vi "Sensor.vi"() -> ()   [LabVIEW 2020]
uses:
  Global_Variable/Global.vi
  Global_Variable/excursion.vi
panel:
  in  "Sensor":T1
  # "扭矩偏移"
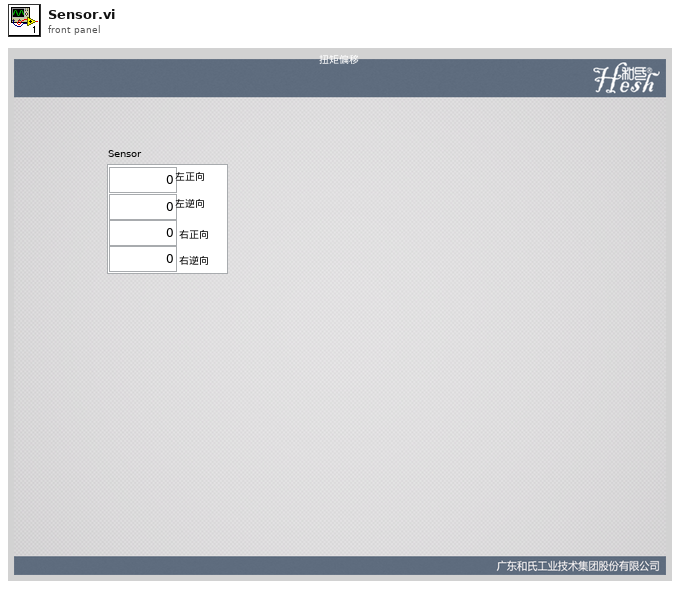
[diagram p1: front panel]
types:
  T1 = cluster{"左正向":dbl, "左逆向":dbl, "右正向":dbl, "右逆向":dbl}
  T2 = typedef "Sensor.ctl" = cluster{"左正向":dbl, "左逆向":dbl, "右正向":dbl, "右逆向":dbl}
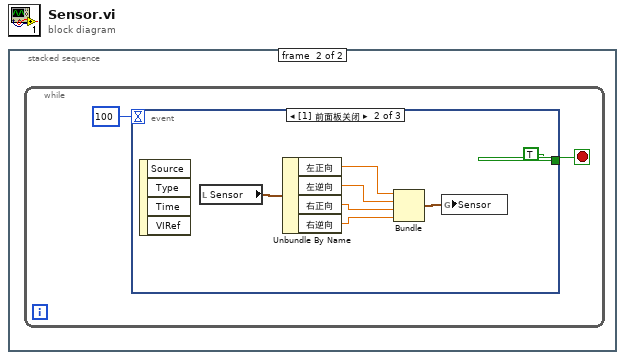
[diagram p0: block diagram]
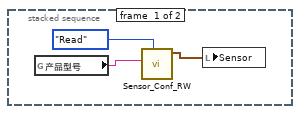
[diagram p2: hidden frame]
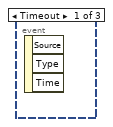
[diagram p3: hidden frame]
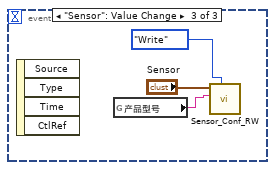
[diagram p4: hidden frame]
diagram:
  n1 = stacked-sequence {
    frame #0 {
      n2 = global read "Global.vi" "产品型号"() -> (w2:string)
      n3 = call "Sensor_Conf_RW.vi"("Mode"=enum16{"Read", "Write"}."Read", "Section"=w2) -> ("Sensor_OUT"=w1:T2)  [unwired: 8 in, 1 out]
      n4 = local write "Sensor"(w1) -> ()
    }
    frame #1 {
      n5 = while {
        stop <- w5 stop-if-true
        n6 = event shown="[1] 前面板关闭" {
          selector: _ -> [_ _ _]
          dyn-events: _ -> [_ _ _]
          timeout: 100 -> [_ _ _]
          tunnel: [_ TRUE _] -> w5
          event Timeout {
            n7 = event-data() -> ()  [unwired: 1 in, 3 out]
          }
          event Panel Close {
            n8 = event-data() -> ()  [unwired: 1 in, 4 out]
            n9 = local read "Sensor"() -> (w11:T1)
            n10 = Unbundle By Name(w11) -> ("左正向"=w10:dbl, "左逆向"=w9:dbl, "右正向"=w8:dbl, "右逆向"=w7:dbl)
            n11 = Bundle("左正向"=w10, "左逆向"=w9, "右正向"=w8, "右逆向"=w7) -> (w6:T1)  [unwired: 1 in]
            n12 = global write "excursion.vi" "Sensor"(w6) -> ()
          }
          event "Sensor": Value Change {
            n13 = event-data() -> ()  [unwired: 1 in, 4 out]
            n14 = global read "Global.vi" "产品型号"() -> (w13:string)
            n15 = call "Sensor_Conf_RW.vi"("Mode"=enum16{"Read", "Write"}."Write", "Section"=w13, "Sensor_IN"="Sensor") -> ()  [unwired: 7 in, 2 out]
          }
        }
      }
    }
  }
